vi "Process Data and Plot XYGraph.vi"(8 "error in (no error)":errorcluster, 9 "Pressure":dbl[](array[numeric]), 10 "Graph":dbl[](array[numeric]), 11 "WaveformGraph in":refnum<vi>) -> (0 "error out":errorcluster)   [LabVIEW 2013, in "main.lvlib"]
uses:
  main.lvlib
  Controls/Enum Variables.ctl
  <vilib>/Analysis/baseanly.llb/Mean (DBL).vi
  <vilib>/Analysis/NI_AALBase.lvlib
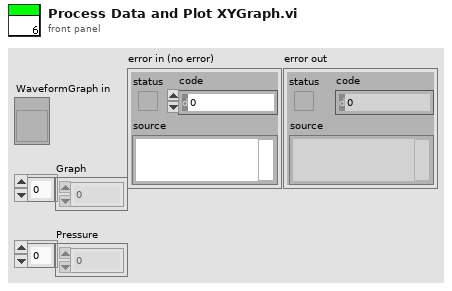
[diagram p1: front panel]
types:
  T1 = typedef "main.lvlib/Enum Variables.ctl" = enum16{"SetAcqFilter", "GetAcqFilter", "Set Filter", "Get Filter", "Set Height", "Get Height", "Set Blue Pressure", "Get Blue Pressure", "Set Red Pressure", "Get Red Pressure", "Init", "Reset Pressure", "Set Red Cursors", "Get Red Cursors", "Set Blue Cursors", "Get Blue Cursors", "Set Language", "Get Language", "Set Active Graphs", "Get ActiveGraphs", "Set Method", "Get Method", "Set Encryption", "Get Encryption", "Set ExcelVersion", "Get ExcelVersion", "Set DICOM Avail", "Get DICOM Avail", "Set DICOM Encode", "Get DICOM Encode", "Set JournalExport", "Get JournalExport", "Set Sequence", "Get Sequence", "Set DAQ Connected", "Get DAQ Connected", "Set Current Graph", "Get Current Graph", "Set General Settings", "Get Hyphenation", "Set Arm Calc Method", "Get Arm Calc Method", "Set Dicom Tags", "Get Dicom Tags", "Set BT Serial", "Get BT Serial", "Set BT Accepted Serials", "Get BT Accepted Serials", "Get BT License", "Set BT License"}
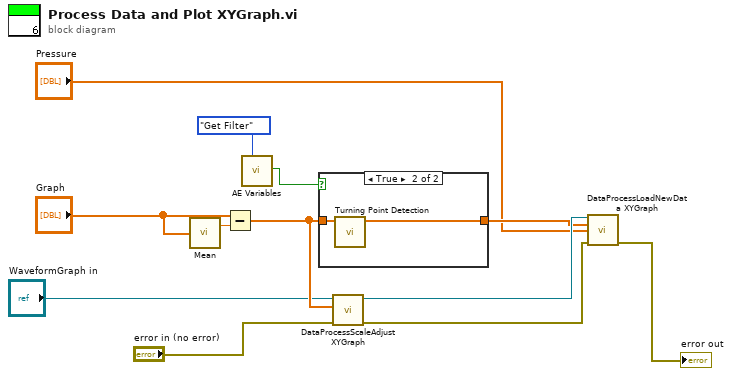
[diagram p0: block diagram]
diagram:
  n1 = call-poly <vilib>:"Mean.vi"("X"="Graph") -> ("mean"=w6:dbl)  [unwired: 1 out]
  n2 = Subtract(x="Graph", y=w6) -> (x-y=w10:dbl[])
  n3 = call "AE Variables.vi"("Action"=Enum_Variables."Get Filter") -> ("BooleanOut"=w12:bool)  [unwired: 11 in, 7 out]
  n4 = case shown="True" w12 {
    tunnel: w10 -> [w13 w15]
    tunnel: [w13 w14] -> w2
    frame False {
    }
    frame True {
      n5 = call "Turning Point Detection.vi"("Input"=w15) -> ("Best BSpline Fit"=w14:dbl[])  [unwired: 9 in, 1 out]
    }
  }
  n6 = call "DataProcessScaleAdjust XYGraph.vi"("error in (no error)"="error in (no error)", 10:"Graph"=w10, 11:"Graph"="WaveformGraph in") -> ("error out"=w3:errorcluster, "reference out"=w11:refnum<vi>)  [unwired: 7 in]
  n7 = call "DataProcessLoadNewData XYGraph.vi"(0:"Graph"=w11, 5:"Graph"=w2, "Pressure"="Pressure", "error in (no error)"=w3) -> ("error out"=→"error out":errorcluster)  [unwired: 10 in, 1 out]
